vi "Process Data.vi"(11 "x":u32) -> (3 "Result":u32)   [LabVIEW 2012]
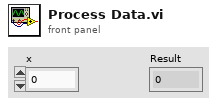
[diagram p1: front panel]
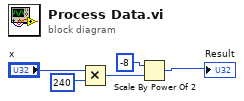
[diagram p0: block diagram]
diagram:
  n1 = Multiply(x="x", y=u32 240) -> (x*y=w3:u32)
  n2 = Scale By Power Of 2(n=-8, x=w3) -> (x*2^n=→"Result":u32)
